vi "Trigger.vi"(8 "error in (no error)":errorcluster, 11 "NIDIO in":refnum<class "NIDIO.lvclass">) -> (0 "error out":errorcluster, 3 "NIDIO out":refnum<class "NIDIO.lvclass">)   [LabVIEW 2015, in "NIDIO.lvclass"]
uses:
  NIDIO.lvclass
  DIO.lvclass
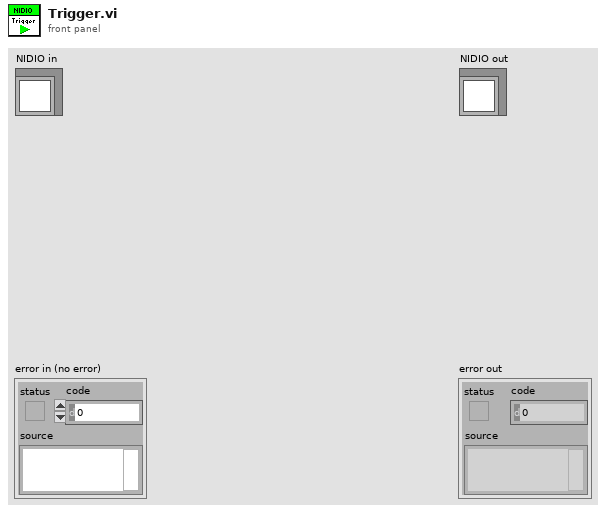
[diagram p1: front panel]
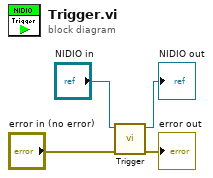
[diagram p0: block diagram]
diagram:
  n1 = call-parent "Trigger.vi"("error in (no error)"="error in (no error)", "DIO in"="NIDIO in") -> ("error out"=→"error out":errorcluster, "DIO out"=→"NIDIO out":refnum<class "NIDIO.lvclass">)  [unwired: 8 in]
